vi "KB-组合.vi"(9 "StartTimer":string, 10 "Barcode":string, 11 "ResultMessage":string[][](array[string])) -> (3 "Data":string[][](array[string]))   [LabVIEW 2015]
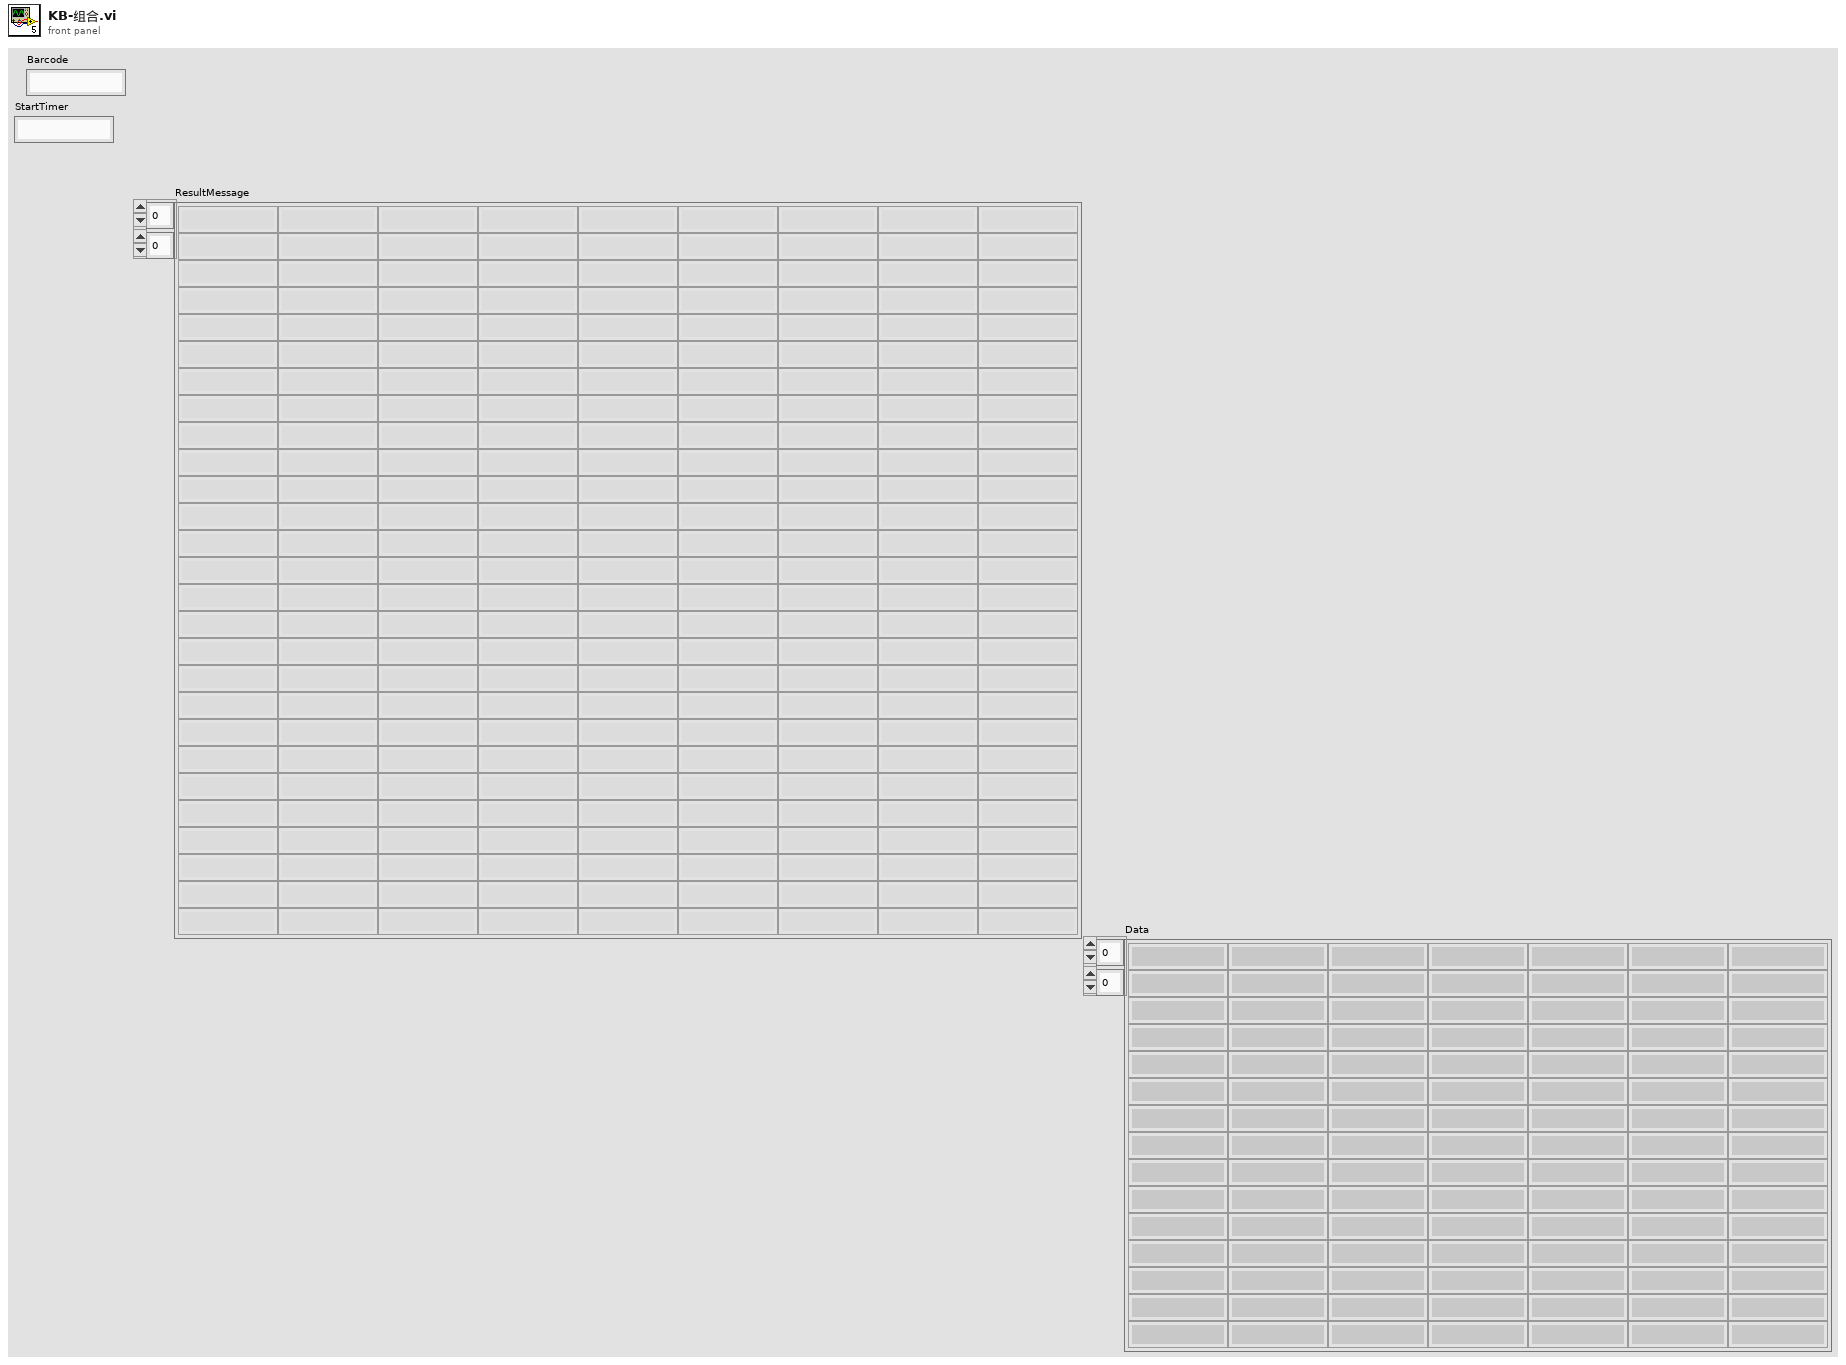
[diagram p1: front panel]
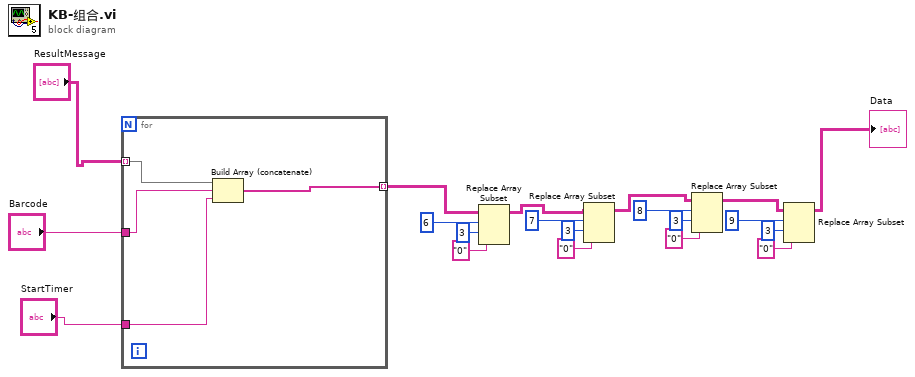
[diagram p0: block diagram]
diagram:
  n1 = for {
    tunnel: "ResultMessage" -> [w24] mode=indexing
    tunnel: "Barcode" -> [w23]
    tunnel: [w22] -> w18 mode=indexing
    tunnel: "StartTimer" -> [w21]
    n2 = Build Array (concatenate)(w24, w23, w21) -> (w22:string[])
  }
  n3 = Replace Array Subset(array=w18, new element="0" ("新元素/子数组"), index (row)=6 ("禁用的索引 (行)"), index (col)=3 ("禁用的索引 (列)")) -> (w5:string[][])
  n4 = Replace Array Subset(array=w5, new element="0" ("新元素/子数组"), index (row)=7 ("禁用的索引 (行)"), index (col)=3 ("禁用的索引 (列)")) -> (w4:string[][])
  n5 = Replace Array Subset(array=w4, new element="0" ("新元素/子数组"), index (row)=8 ("禁用的索引 (行)"), index (col)=3 ("禁用的索引 (列)")) -> (w3:string[][])
  n6 = Replace Array Subset(array=w3, new element="0" ("新元素/子数组"), index (row)=9 ("禁用的索引 (行)"), index (col)=3 ("禁用的索引 (列)")) -> (→"Data":string[][])
